vi "39 GPS Array to String (x64-2018).vi"(0 "Input String":string) -> (1 "Output String":string, 2 "Code valid?":bool)   [LabVIEW 2017]
panel:
  out "Array Size":dbl
  out "End of String?":bool
  out "End of String Numb":dbl
  out "Array of Strings":string[](array[string])
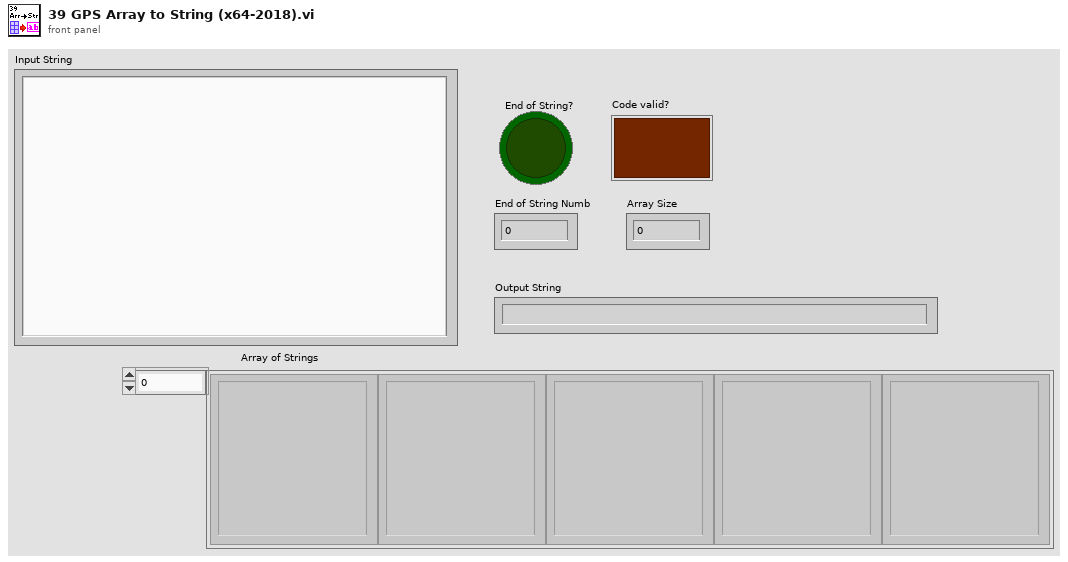
[diagram p1: front panel]
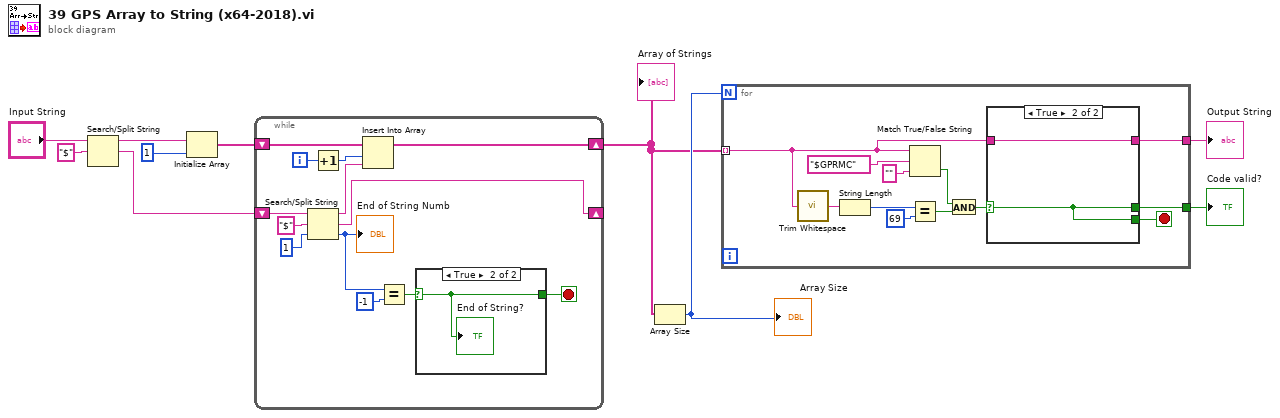
[diagram p0: block diagram]
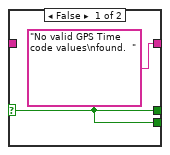
[diagram p2: hidden frame]
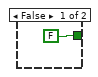
[diagram p3: hidden frame]
diagram:
  n1 = Search/Split String(string="Input String", search string/char (-)="$") -> (substring before match=w8:string, match + rest of string=w6:string)  [unwired: 1 in, 1 out]
  n2 = Initialize Array(w8, 1) -> (w5:string[])
  n3 = while {
    shift-right: [w16] -> w3
    shift-left: w5 -> [w15]
    shift-right: [w11] -> _
    shift-left: w6 -> [w14]
    i -> [w13]
    stop <- w12 stop-if-true
    n4 = Search/Split String(string=w14, search string/char (-)="$", offset (0)=1) -> (substring before match=w20:string, match + rest of string=w11:string, offset of match=w19:i32)
    "End of String Numb" <- w19
    n5 = Increment(x=w13) -> (x+1=w21:i32)
    n6 = Insert Into Array(array=w15, index=w21, new element=w20) -> (w16:string[])
    n7 = Equal?(x=w19, y=-1) -> (x = y?=w17:bool)
    n8 = case shown="True" w17 {
      selector: w17 -> [_ w25]
      tunnel: [FALSE w25] -> w12
      frame False {
      }
      frame True {
        "End of String?" <- w25
      }
    }
  }
  "Array of Strings" <- w3
  n9 = Array Size(array=w3) -> (size(s)=w4:i32)
  "Array Size" <- w4
  n10 = for {
    N: w4 -> [_]
    tunnel: w3 -> [w27] mode=indexing
    tunnel: [w34] -> w2
    tunnel: [w33] -> w1
    stop <- w35 stop-if-true
    n11 = call <vilib>:"Trim Whitespace.vi"("string"=w27) -> ("trimmed string"=w26:string)  [unwired: 1 in]
    n12 = String Length(string=w26) -> (length=w32:i32)
    n13 = Match True/False String(2:"", 3:"$GPRMC", 4:w27) -> (0:w30:bool)  [unwired: 1 out]
    n14 = Equal?(x=w32, y=69) -> (x = y?=w29:bool)
    n15 = And(x=w30, y=w29) -> (x .and. y?=w28:bool)
    n16 = case shown="True" w28 {
      selector: w28 -> [w38 w40]
      tunnel: w27 -> [_ w41]
      tunnel: ["No valid GPS Time code values\nfound.  " w41] -> w34
      tunnel: [w38 w40] -> w33
      tunnel: [w38 w40] -> w35
      frame False {
      }
      frame True {
      }
    }
  }
  "Output String" <- w2
  "Code valid?" <- w1
